vi "RT Video Output Setup.vi"() -> ()   [LabVIEW 2015]
doc: "The Video Setup Example VI shows different resolutions that could be support for PXI Video Out. You must have a RT target with an i815 graphics chipset to run this example."
panel:
  in  "Stop":bool
  in  "Video Mode":T1={"Screen Area"=1, "Color Depth"=0, "Refresh Frequency"=0} caption="Video Mode Settings" {"Refresh Frequency" items=["60 Hz", "70 Hz", "72 Hz", "75 Hz", "85 Hz"]; "Color Depth" items=["8 bits", "15 bits", "16 bits", "24 bits", "32 bits"]; "Screen Area" items=["Text Mode", "640 x 480", "800 x 600", "1024 x 768", "1280 x 1024"]}
  # "Overview: Demonstrates how to use the IMAQ Video Out Display Mode function to change how the video out for a Real-Time target is displayed on a monitor, and how to use IMAQ Video RT Out to display the image on the monitor.\nRequirements: Vision Development Software, LabVIEW Real-Time, Real-Time target with i815 graphics chipset.\nInstructions:\n1. Open a New LabVIEW Project. Select to Add this VI to the project when prompted.\n2. Right click on the Project in the tree and select New>>Targets and Devices...\n3. Select the target you want to run this example with, and click OK.\n4. Drag this VI from My Computer to the target in the tree.\n5. Double click on the example under the target, and run the VI.\n6. Change the Video Mode Settings to see how the image displayed on the monitor is affected.\nNOTE: The last Video Mode Settings used by this VI will be what the target uses until they are changed or the target is rebooted."
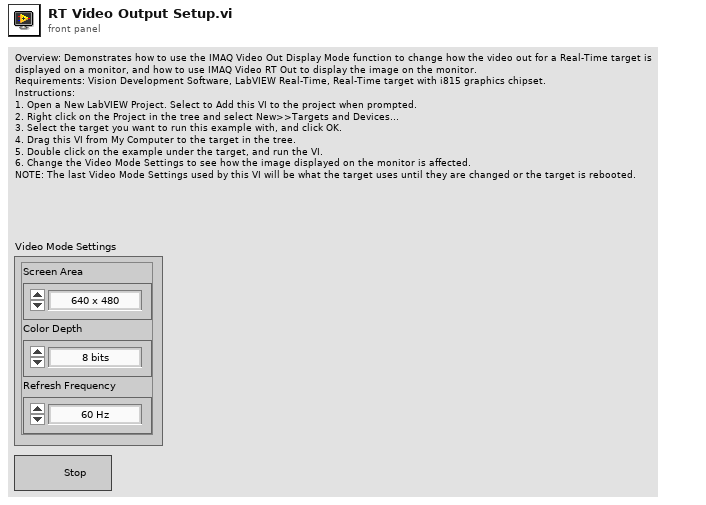
[diagram p1: front panel]
types:
  T1 = cluster{"Screen Area":u32, "Color Depth":u32, "Refresh Frequency":u32}
  T2 = typedef "Image Type" = u32
  T3 = typedef "IMAQ Image.ctl" = refnum<image>
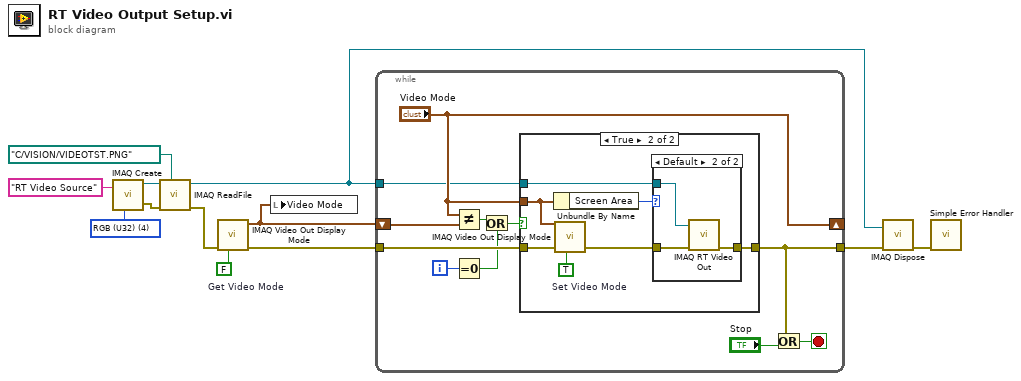
[diagram p0: block diagram]
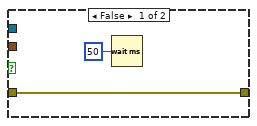
[diagram p2: hidden frame]
diagram:
  w5 = T2 4 items=["Grayscale (U8)", "Grayscale (I16)", "Grayscale (SGL)", "Complex (CSG)", "RGB (U32)", "HSL (U32)", "RGB (U64)", "Grayscale (U16)"] ("Image Type")
  w12 = FALSE  # Get Video Mode
  n1 = call "IMAQ Create"("Image Name"="RT Video Source", "Image Type"=w5) -> ("New Image"=w8:T3, "error out"=w4:errorcluster)  [unwired: 2 in, 1 out]
  n2 = call "IMAQ ReadFile"("File Path"=path "C:/VISION/VIDEOTST.PNG", "error in (no error)"=w4, "Image"=w8) -> ("error out"=w2:errorcluster, "Image Out"=w1:T3)  [unwired: 2 in, 5 out]
  n3 = call "IMAQ Video Out Display Mode"("Get/Set Status? (Set)"=w12, "error in (no error)"=w2) -> ("error out"=w9:errorcluster, "Video Mode Out"=w3:T1)  [unwired: 1 in, 7 out]
  n4 = local write "Video Mode"(w3) -> ()
  n5 = while {
    tunnel: w9 -> [w23]
    tunnel: [w19] -> w11
    tunnel: w1 -> [w20]
    shift-right: ["Video Mode"] -> _
    shift-left: w3 -> [w22]
    i -> [w15]
    stop <- w17 stop-if-true
    n6 = Not Equal?(x="Video Mode", y=w22) -> (x != y?=w16:bool)
    n7 = Equal To 0?(x=w15) -> (x = 0?=w14:bool)
    n8 = Or(x=w16, y=w14) -> (x .or. y?=w13:bool)
    n9 = case shown="True" w13 {
      tunnel: w23 -> [w25 w32]
      tunnel: [w25 w29] -> w19
      tunnel: w20 -> [_ w27]
      tunnel: "Video Mode" -> [_ w26]
      frame False {
        n10 = Wait (ms)(milliseconds to wait=u32 50) -> ()  [unwired: 1 out]
      }
      frame True {
        w31 = TRUE  # Set Video Mode
        n11 = Unbundle By Name(w26) -> ("Screen Area"=w28:u32)
        n12 = call "IMAQ Video Out Display Mode"("Get/Set Status? (Set)"=w31, "error in (no error)"=w32, "Video Mode"=w26) -> ("error out"=w30:errorcluster)  [unwired: 8 out]
        n13 = case shown="Default" w28 {
          tunnel: w30 -> [w33 w35]
          tunnel: [w33 w36] -> w29
          tunnel: w27 -> [_ w34]
          frame 0 {
            # "Text Mode"
          }
          frame Default {
            n14 = call "IMAQ RT Video Out"("error in (no error)"=w35, "Image"=w34) -> ("error out"=w36:errorcluster)  [unwired: 1 in, 8 out]
          }
        }
      }
    }
    n15 = Or(x=w19, y="Stop") -> (x .or. y?=w17:bool)
  }
  n16 = call "IMAQ Dispose"("Image"=w1, "error in (no error)"=w11) -> ("error out"=w10:errorcluster)  [unwired: 1 in, 3 out]
  n17 = call <vilib>:"Simple Error Handler.vi"("error in (no error)"=w10) -> ()  [unwired: 1 in, 8 out]
